vi "configuration UI.vi"() -> ()   [LabVIEW 2013, in "user tag bus module editor node.lvclass"]
uses:
  user tag bus module editor node.lvclass
  <vilib>/NI/Configuration Framework/Node/NodeRef.ctl
  <vilib>/NI/Configuration Framework/Node/NISE_CEF_Node.lvclass
  <vilib>/NI/AMC/Message Queue.ctl
  <vilib>/NI/AMC/Message.ctl
  <vilib>/NI/Tools/Keyed Array/KeyedArray.ctl
  <vilib>/NI/Configuration Framework/Node/UserEventRef.ctl
  <vilib>/NI/Configuration Framework/Controls/EventCluster.ctl
  <vilib>/NI/Configuration Framework/Node/StopEvent.ctl
  <vilib>/NI/Configuration Framework/Node/RefreshUIEvent.ctl
  <vilib>/NI/Configuration Framework/Node/CacheState.ctl
  <vilib>/NI/Configuration Framework/Node/NodeChangeEvent.ctl
  module/configuration/state module configuration.ctl
  <vilib>/NI/Tag Bus Module Framework/channel/TBM channel.lvclass
  user tag bus module editor node.lvclass/user tag bus module editor node.ctl
  module/configuration/user tag bus module configuration.lvclass/user tag bus module configuration.ctl
  module/configuration/user tag bus module configuration.lvclass
  <vilib>/NI/Tag Bus Data Framework/Configuration Editor/Classes/Engine Parent/Engine Parent Editor Node.lvclass
  <vilib>/NI/Tools/Keyed Array/Tools_KeyedArray.lvlib
  <vilib>/NI/AMC/AMC.lvlib
  <vilib>/NI/Configuration Framework/NISE_CEF_TreeControl.lvlib
panel:
  in  "node change":T1
  in  "cache state":T2
  in  "refresh UI":T3
  in  "stop event":T4
  in  "Tab Control":enum32{"Static State Configuration"}(tab)
  in  "Output Tag":u16(ring)
  in  "Input Tag":u16(ring)
  in  "Initial State":u8
  in  "user event":T5
  in  "main queue":T6
  in  "node ref":T7
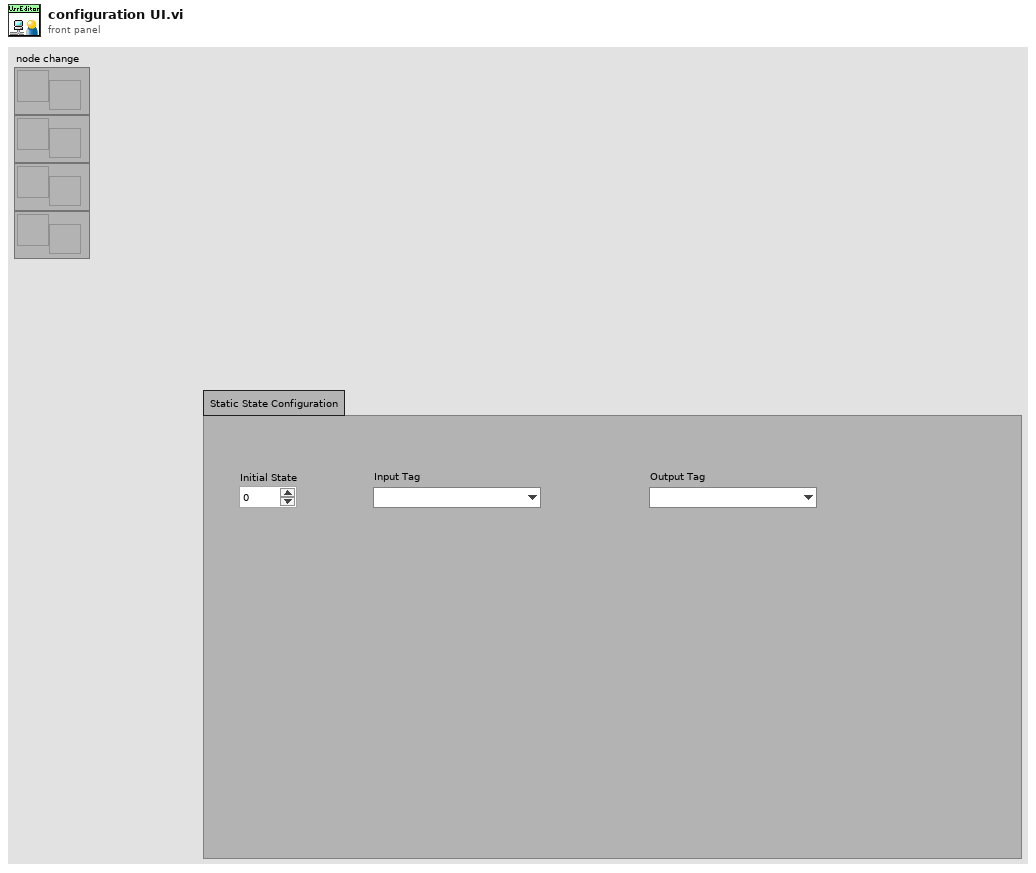
[diagram p1: front panel]
types:
  T1 = typedef "NISE_CEF_Node.lvclass/NodeChangeEvent.ctl" = refnum<user-event>
  T2 = typedef "NISE_CEF_Node.lvclass/CacheState.ctl" = refnum<user-event>
  T3 = typedef "NISE_CEF_Node.lvclass/RefreshUIEvent.ctl" = refnum<user-event>
  T4 = typedef "NISE_CEF_Node.lvclass/StopEvent.ctl" = refnum<user-event>
  T5 = typedef "NISE_CEF_Node.lvclass/UserEventRef.ctl" = refnum<user-event>
  T6 = typedef "AMC.lvlib/Message Queue.ctl" = refnum<queue>
  T7 = typedef "NISE_CEF_Node.lvclass/NodeRef.ctl" = refnum<data-value>
  T8 = typedef "user tag bus module configuration.lvclass/state module configuration.ctl" = cluster{"fixed input":refnum<class "TBM channel.lvclass">, "fixed output":refnum<class "TBM channel.lvclass">, "initial state":u8}
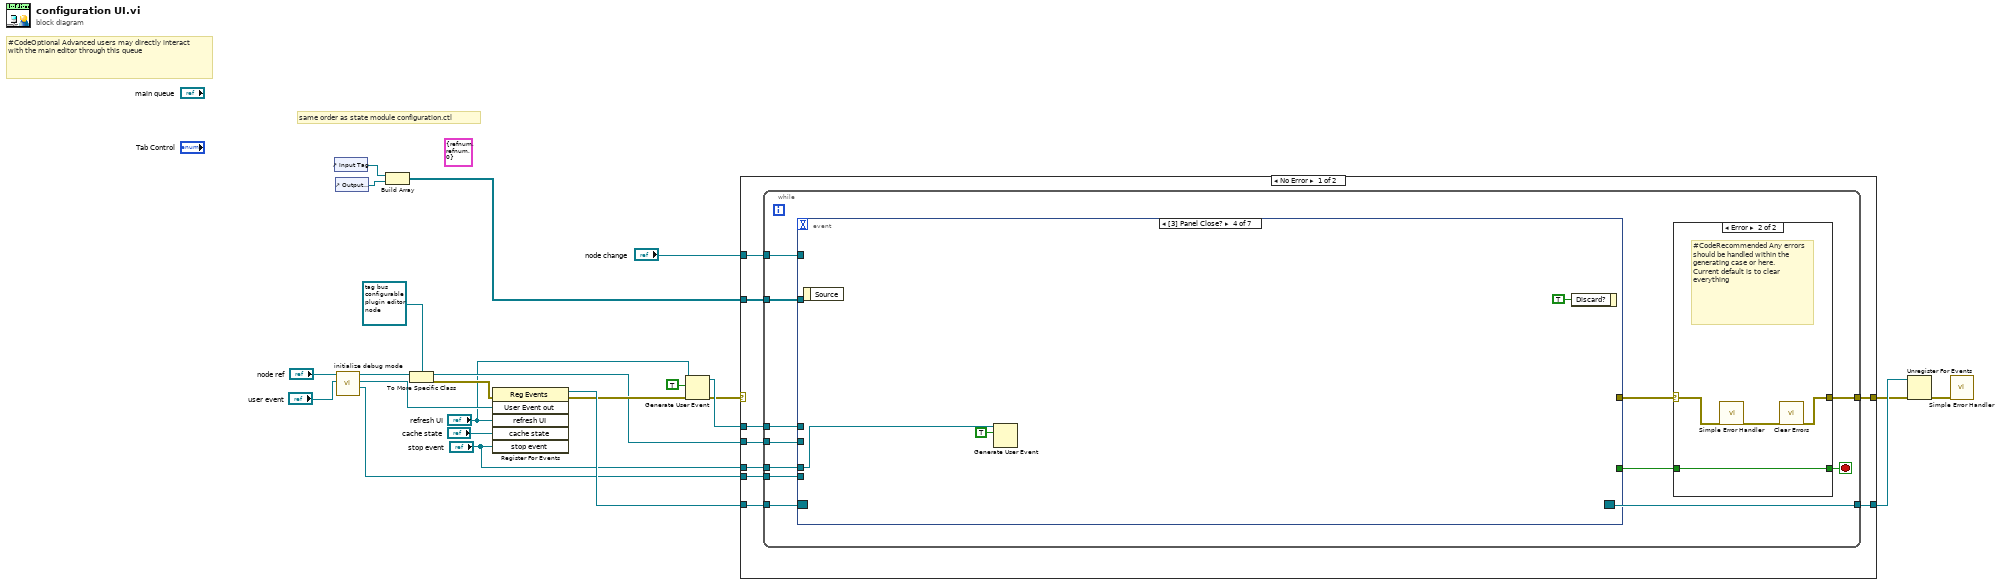
[diagram p0: block diagram]
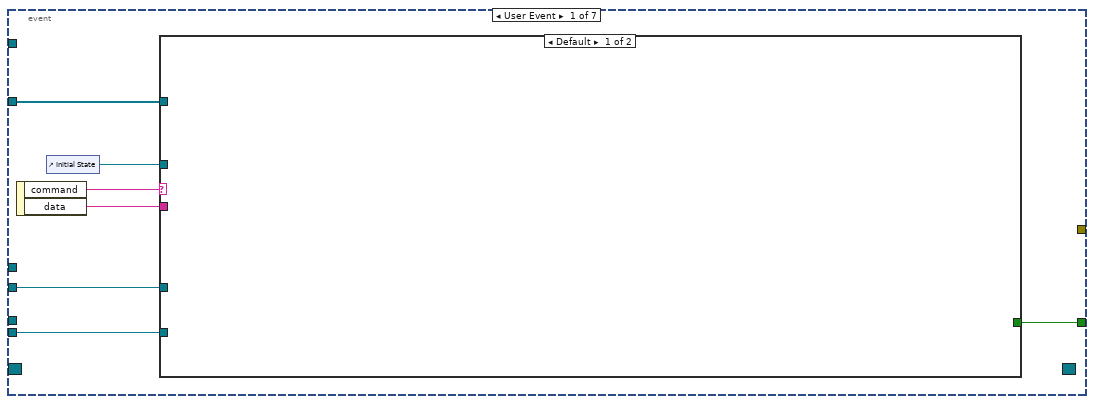
[diagram p3: hidden frame]
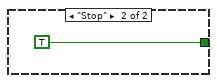
[diagram p4: hidden frame]
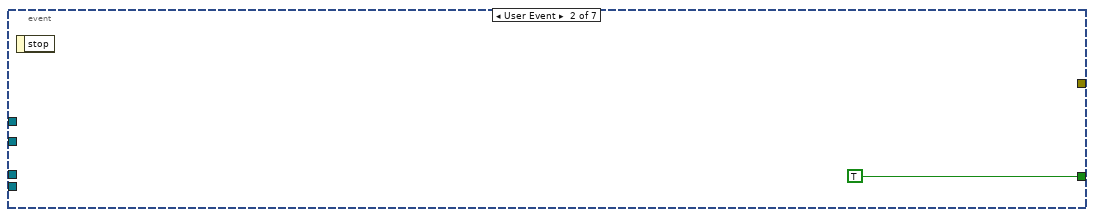
[diagram p5: hidden frame]
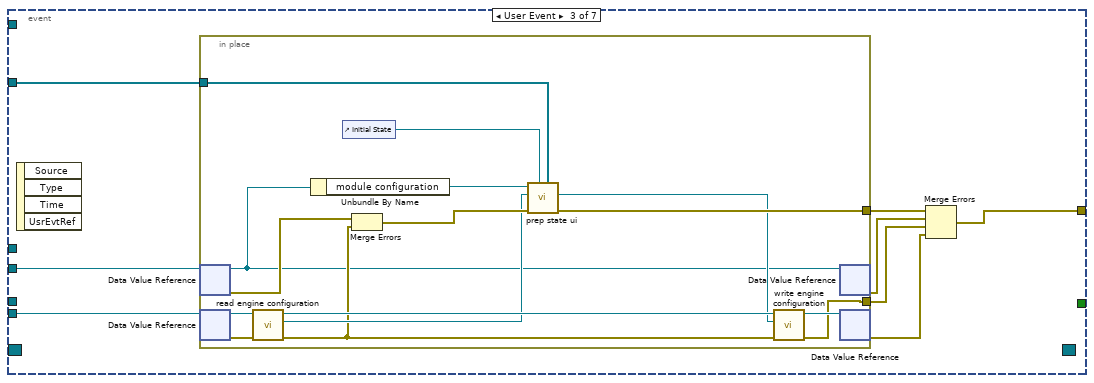
[diagram p6: hidden frame]
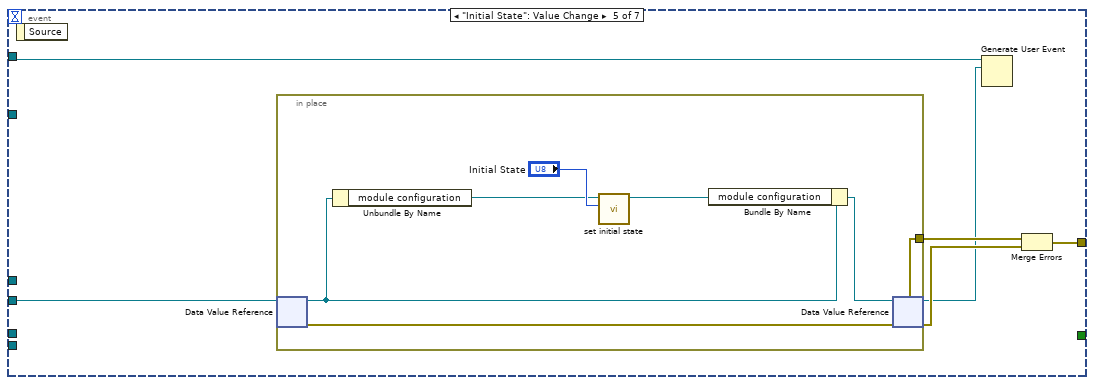
[diagram p7: hidden frame]
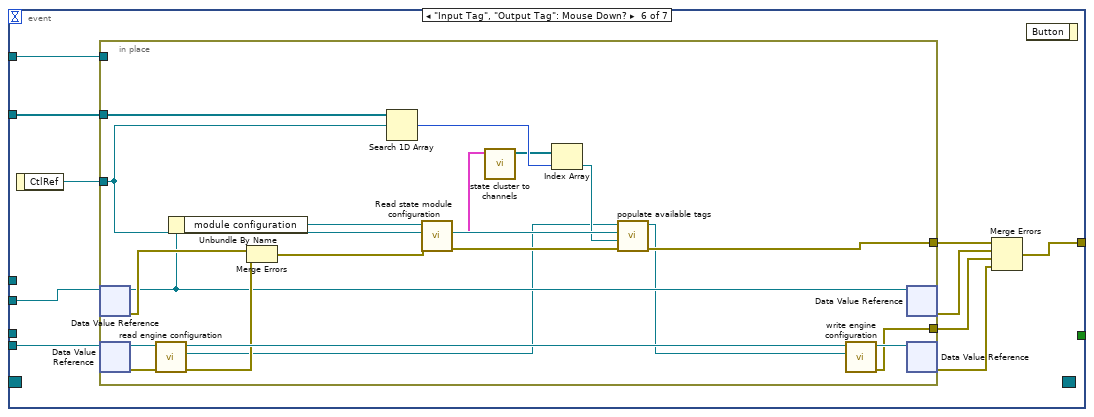
[diagram p8: hidden frame]
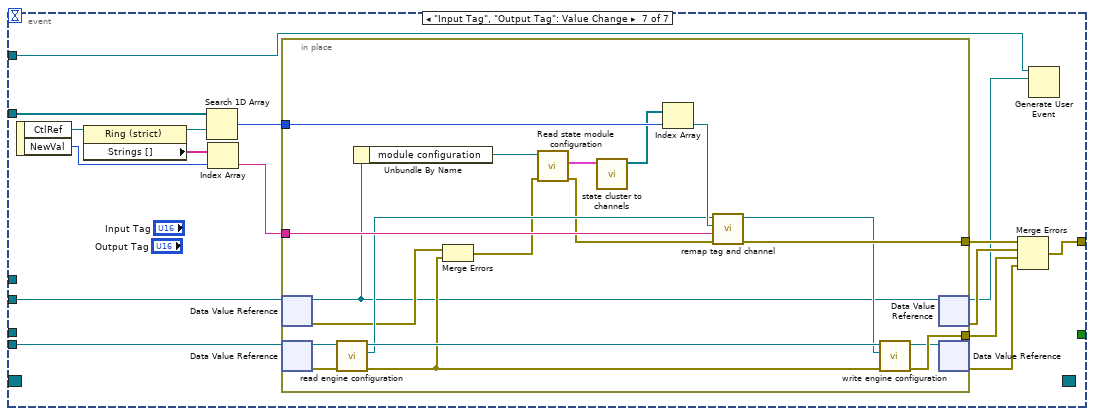
[diagram p9: hidden frame]
diagram:
  (unwired) T8 {"fixed input"=refnum, "fixed output"=refnum, "initial state"=0} ("state module configuration")
  # "same order as state module configuration.ctl"
  # "#CodeOptional Advanced users may directly interact with the main editor through this queue"
  n1 = control-ref of="Input Tag"() -> (w12:refnum<vi>)
  n2 = control-ref of="Output Tag"() -> (w13:refnum<vi>)
  n3 = call "initialize debug mode.vi"("User Event in"="user event", "editor node in"="node ref") -> ("engine"=w14:refnum<data-value>, "User Event out"=w10:T5, "editor node out"=w17:T7)  [unwired: 7 in]
  n4 = Build Array(w12, w13) -> (w11:refnum<vi>[])
  n5 = To More Specific Class(target class=refnum<data-value> refnum ("data value reference"), reference=w17) -> (specific class reference=w9:refnum<data-value>, error out=w8:errorcluster)  [unwired: 1 in]
  n6 = register-events(error in=w8, w10, "refresh UI", "cache state", "stop event") -> (reference out=w23:refnum<event-registration>, error out=w19:errorcluster)  [unwired: 1 in]
  n7 = Generate User Event(user event="refresh UI", event data cluster=TRUE ("event data"), error in=w19) -> (user event out=w7:T3, error out=w1:errorcluster)  [unwired: 1 in]
  n8 = case shown="No Error" w1 {
    selector: w1 -> [_ w164]
    tunnel: w23 -> [w32 w163]
    tunnel: [w31 w163] -> w22
    tunnel: [w30 w164] -> w21
    tunnel: w14 -> [w29 _]
    tunnel: w11 -> [w28 _]
    tunnel: w9 -> [w27 _]
    tunnel: w7 -> [w26 _]
    tunnel: "node change" -> [w25 _]
    tunnel: "stop event" -> [w24 _]
    frame No Error {
      n9 = while {
        tunnel: w32 -> [w44]
        tunnel: [w43] -> w31
        tunnel: w27 -> [w39]
        tunnel: w29 -> [w38]
        tunnel: w28 -> [w37]
        tunnel: w26 -> [w36]
        tunnel: w25 -> [w34]
        tunnel: w24 -> [w33]
        tunnel: [w40] -> w30
        stop <- w41 stop-if-true
        n10 = event shown="[3] Panel Close?" {
          selector: w44 -> [_ _ _ _ _ _ _]
          dyn-events: [_ _ _ _ _ _ _] -> w43
          timeout: _ -> [_ _ _ _ _ _ _]
          tunnel: [w57 TRUE _ _ _ _ _] -> w35
          tunnel: [_ _ w67 _ w90 w104 w135] -> w42
          tunnel: w39 -> [w55 _ w66 _ w91 w102 w133]
          tunnel: w38 -> [w54 _ w65 _ _ w103 w134]
          tunnel: w37 -> [w51 _ w64 _ _ w106 w139]
          tunnel: w36 -> [_ _ _ _ _ _ _]
          tunnel: w34 -> [_ _ _ _ w86 w98 w128]
          tunnel: w33 -> [_ _ _ w84 _ _ _]
          event User Event {
            n11 = event-data() -> ("command"=w56:string, "data"=w53:string)  [unwired: 1 in]
            n12 = control-ref of="Initial State"() -> (w52:refnum<vi>)
            n13 = case shown="Default" w56 {
              tunnel: [_ TRUE] -> w57
              tunnel: w54 -> [_ _]
              tunnel: w55 -> [_ _]
              tunnel: w53 -> [_ _]
              tunnel: w52 -> [_ _]
              tunnel: w51 -> [_ _]
              frame Default {
              }
              frame "Stop" {
              }
            }
          }
          event User Event {
            n14 = event-data() -> ()  [unwired: 1 in, 1 out]
          }
          event User Event {
            n15 = event-data() -> ()  [unwired: 1 in, 4 out]
            n16 = in-place {
              in-place-border: [w82] -> w63
              in-place-border: w64 -> [w81]
              in-place-border: [w78] -> w60
              n17 = in-place-dvr #1(w66) -> (w70:refnum<class "user tag bus module editor node.lvclass">, w71:errorcluster)
              n18 = in-place-dvr #2(w65) -> (w77:refnum<class "Engine Parent Editor Node.lvclass">, w76:errorcluster)
              n19 = call <vilib>:"read engine configuration.vi"("error in"=w76, "Engine Parent Editor Node in"=w77) -> ("error out"=w72:errorcluster, "engine configuration"=w73:refnum<class "engine configuration.lvclass">, "Engine Parent Editor Node out"=w75:refnum<class "Engine Parent Editor Node.lvclass">)  [unwired: 7 in]
              n20 = Unbundle By Name(w70) -> ("module configuration"=w69:refnum<class "user tag bus module configuration.lvclass">)
              n21 = control-ref of="Initial State"() -> (w68:refnum<vi>)
              n22 = Merge Errors(w71, w72) -> (w80:errorcluster)
              n23 = call "prep state ui.vi"("tag references"=w81, "Initial State"=w68, "error in"=w80, "engine configuration in"=w73, "user tag bus module configuration in"=w69) -> ("error out"=w82:errorcluster, "engine configuration out"=w74:refnum<class "engine configuration.lvclass">)  [unwired: 5 in]
              n24 = call <vilib>:"write engine configuration.vi"("error in"=w72, "engine configuration"=w74, "Engine Parent Editor Node in"=w75) -> ("error out"=w78:errorcluster, "Engine Parent Editor Node out"=w79:refnum<class "Engine Parent Editor Node.lvclass">)  [unwired: 7 in]
              n25 = in-place-dvr #1(w70) -> (w61:errorcluster)  [unwired: 1 out]
              n26 = in-place-dvr #2(w79) -> (w62:errorcluster)  [unwired: 1 out]
            }
            n27 = Merge Errors(w63, w61, w60, w62) -> (w67:errorcluster)
          }
          event Panel Close? {
            n28 = event-data() -> ()  [unwired: 1 in, 1 out]
            n29 = Generate User Event(user event=w84, event data cluster=TRUE ("event data")) -> ()  [unwired: 2 in, 2 out]
            n30 = event-data("Discard?"=TRUE) -> ()  [unwired: 1 in, 1 out]
          }
          event "Initial State": Value Change {
            n31 = event-data() -> ()  [unwired: 1 in, 1 out]
            n32 = in-place {
              in-place-border: [w96] -> w89
              n33 = in-place-dvr #3(w91) -> (w95:refnum<class "user tag bus module editor node.lvclass">, w96:errorcluster)
              n34 = Unbundle By Name(w95) -> ("module configuration"=w93:refnum<class "user tag bus module configuration.lvclass">)
              n35 = call "set initial state.vi"("state module configuration.initial state"="Initial State", "tag bus configurable plugin module configuration in"=w93) -> ("tag bus configurable plugin module configuration out"=w92:refnum<class "user tag bus module configuration.lvclass">)  [unwired: 9 in]
              n36 = Bundle By Name(cluster=w95, "module configuration"=w92) -> (w94:refnum<class "user tag bus module editor node.lvclass">)
              n37 = in-place-dvr #3(w94) -> (w87:refnum<data-value>, w88:errorcluster)
            }
            n38 = Generate User Event(user event=w86, event data cluster=w87) -> ()  [unwired: 2 in, 2 out]
            n39 = Merge Errors(w89, w88) -> (w90:errorcluster)
          }
          event "Input Tag", "Output Tag": Mouse Down? {
            n40 = event-data() -> ("CtlRef"=w105:refnum<vi>)  [unwired: 1 in]
            n41 = in-place {
              in-place-border: [w127] -> w107
              in-place-border: w106 -> [w126]
              in-place-border: w105 -> [w125]
              in-place-border: [w112] -> w100
              in-place-border: w98 -> [_]
              n42 = in-place-dvr #4(w102) -> (w111:refnum<class "user tag bus module editor node.lvclass">, w113:errorcluster)
              n43 = in-place-dvr #5(w103) -> (w118:refnum<class "Engine Parent Editor Node.lvclass">, w115:errorcluster)
              n44 = call <vilib>:"read engine configuration.vi"("error in"=w115, "Engine Parent Editor Node in"=w118) -> ("error out"=w114:errorcluster, "engine configuration"=w108:refnum<class "engine configuration.lvclass">, "Engine Parent Editor Node out"=w117:refnum<class "Engine Parent Editor Node.lvclass">)  [unwired: 7 in]
              n45 = Unbundle By Name(w111) -> ("module configuration"=w110:refnum<class "user tag bus module configuration.lvclass">)
              n46 = Merge Errors(w113, w114) -> (w119:errorcluster)
              n47 = Search 1D Array(1D array=w126, element=w125) -> (index of element=w124:i32)  [unwired: 1 in]
              n48 = call "Read state module configuration.vi"("error in"=w119, "user tag bus module configuration In"=w110) -> ("error out"=w120:errorcluster, "state module configuration"=w121:T8)  [unwired: 7 in, 1 out]
              n49 = call "state cluster to channels.vi"("state module configuration"=w121) -> ("channels"=w123:refnum<class "TBM channel.lvclass">[])  [unwired: 10 in]
              n50 = Index Array(array=w123, index=w124) -> (element=w122:refnum<class "TBM channel.lvclass">)
              n51 = call "populate available tags.vi"("error in"=w120, "channel"=w122, "CtlRef"=w125, "engine configuration in"=w108) -> ("error out"=w127:errorcluster, "engine configuration out"=w109:refnum<class "engine configuration.lvclass">)  [unwired: 6 in]
              n52 = call <vilib>:"write engine configuration.vi"("engine configuration"=w109, "Engine Parent Editor Node in"=w117) -> ("error out"=w112:errorcluster, "Engine Parent Editor Node out"=w116:refnum<class "Engine Parent Editor Node.lvclass">)  [unwired: 8 in]
              n53 = in-place-dvr #4(w111) -> (w101:errorcluster)  [unwired: 1 out]
              n54 = in-place-dvr #5(w116) -> (w99:errorcluster)  [unwired: 1 out]
            }
            n55 = Merge Errors(w107, w101, w100, w99) -> (w104:errorcluster)
            n56 = event-data() -> ()  [unwired: 2 in, 1 out]
          }
          event "Input Tag", "Output Tag": Value Change {
            n57 = event-data() -> ("CtlRef"=w143:refnum<vi>, "NewVal"=w137:u16)  [unwired: 1 in]
            n58 = property on="Property Node" class="Ring (strict)"(reference=w143) -> (reference out=w138:refnum<vi>, "Strings []"=w142:string[])  [unwired: 1 in, 1 out]
            n59 = Search 1D Array(1D array=w139, element=w138) -> (index of element=w136:i32)  [unwired: 1 in]
            n60 = Index Array(array=w142, index=w137) -> (element=w140:string)
            n61 = in-place {
              in-place-border: [w162] -> w141
              in-place-border: w140 -> [w161]
              in-place-border: w136 -> [w160]
              in-place-border: [w155] -> w132
              n62 = in-place-dvr #6(w133) -> (w144:refnum<class "user tag bus module editor node.lvclass">, w149:errorcluster)
              n63 = in-place-dvr #7(w134) -> (w157:refnum<class "Engine Parent Editor Node.lvclass">, w156:errorcluster)
              n64 = call <vilib>:"read engine configuration.vi"("error in"=w156, "Engine Parent Editor Node in"=w157) -> ("error out"=w150:errorcluster, "engine configuration"=w152:refnum<class "engine configuration.lvclass">, "Engine Parent Editor Node out"=w153:refnum<class "Engine Parent Editor Node.lvclass">)  [unwired: 7 in]
              n65 = Unbundle By Name(w144) -> ("module configuration"=w147:refnum<class "user tag bus module configuration.lvclass">)
              n66 = Merge Errors(w149, w150) -> (w148:errorcluster)
              n67 = call "Read state module configuration.vi"("error in"=w148, "user tag bus module configuration In"=w147) -> ("error out"=w146:errorcluster, "state module configuration"=w145:T8)  [unwired: 7 in, 1 out]
              n68 = call "state cluster to channels.vi"("state module configuration"=w145) -> ("channels"=w159:refnum<class "TBM channel.lvclass">[])  [unwired: 10 in]
              n69 = Index Array(array=w159, index=w160) -> (element=w158:refnum<class "TBM channel.lvclass">)
              n70 = call "remap tag and channel.vi"("error in"=w146, "tag name"=w161, "channel"=w158, "engine configuration in"=w152) -> ("error out"=w162:errorcluster, "engine configuration out"=w151:refnum<class "engine configuration.lvclass">)  [unwired: 6 in]
              n71 = call <vilib>:"write engine configuration.vi"("error in"=w150, "engine configuration"=w151, "Engine Parent Editor Node in"=w153) -> ("error out"=w155:errorcluster, "Engine Parent Editor Node out"=w154:refnum<class "Engine Parent Editor Node.lvclass">)  [unwired: 7 in]
              n72 = in-place-dvr #6(w144) -> (w129:refnum<data-value>, w131:errorcluster)
              n73 = in-place-dvr #7(w154) -> (w130:errorcluster)  [unwired: 1 out]
            }
            n74 = Merge Errors(w141, w131, w132, w130) -> (w135:errorcluster)
            n75 = Generate User Event(user event=w128, event data cluster=w129) -> ()  [unwired: 2 in, 2 out]
          }
        }
        n76 = case shown="Error" w42 {
          selector: w42 -> [w45 w49]
          tunnel: [w46 w50] -> w41
          tunnel: w35 -> [w46 w50]
          tunnel: [w45 w47] -> w40
          frame No Error {
          }
          frame Error {
            # "#CodeRecommended Any errors should be handled within the generating case or here. Current default is to clear everything"
            n77 = call <vilib>:"Simple Error Handler.vi"("error in (no error)"=w49) -> ("error out"=w48:errorcluster)  [unwired: 4 in, 4 out]
            n78 = call <vilib>:"Clear Errors.vi"("error in (no error)"=w48) -> ("error out"=w47:errorcluster)  [unwired: 6 in]
          }
        }
      }
    }
    frame Error {
    }
  }
  n79 = Unregister For Events(event registration refnum=w22, error in=w21) -> (error out=w18:errorcluster)
  n80 = call <vilib>:"Simple Error Handler.vi"("error in (no error)"=w18) -> ()  [unwired: 4 in, 5 out]
